vi "Left_to_Right_voltage.vi"(1 "left":dbl) -> (0 "right":dbl)   [LabVIEW 2009]
uses:
  <vilib>/gmath/NI_Gmath.lvlib
panel:
  in  "Left / Right Correlation":cluster{"right":dbl, "left":dbl}[](array[cluster])=[{"right"=0.0, "left"=0.0}, {"right"=0.52, "left"=0.5}, {"right"=0.79, "left"=0.75}, {"right"=1.02, "left"=1.0}, {"right"=1.27, "left"=1.25}, {"right"=1.52, "left"=1.5}, {"right"=1.77, "left"=1.75}, {"right"=2.0, "left"=2.0}, {"right"=2.25, "left"=2.25}, {"right"=2.5, "left"=2.5}, {"right"=2.75, "left"=2.75}, {"right"=3.0, "left"=3.0}, {"right"=3.23, "left"=3.25}, {"right"=3.48, "left"=3.5}, {"right"=3.71, "left"=3.75}, {"right"=3.96, "left"=4.0}, {"right"=4.22, "left"=4.25}, {"right"=4.45, "left"=4.5}, {"right"=4.56, "left"=4.75}, {"right"=4.58, "left"=5.0}]
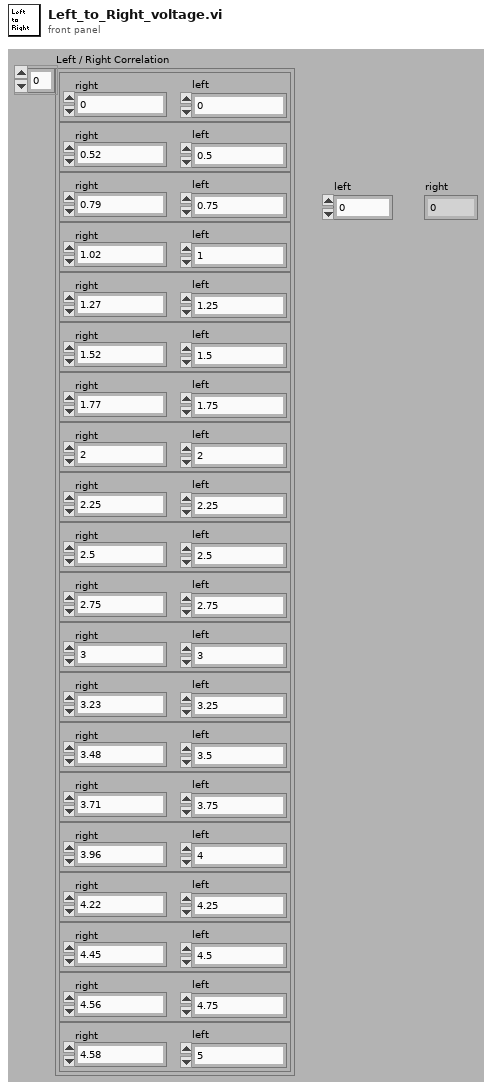
[diagram p1: front panel]
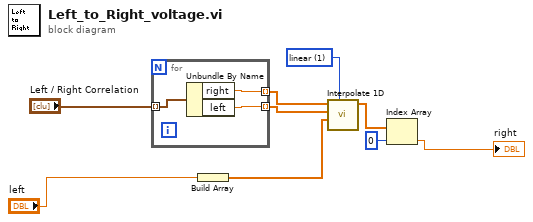
[diagram p0: block diagram]
diagram:
  w9 = 1 items=["nearest", "linear", "spline", "cubic Hermite", "Lagrange"] ("method")
  n1 = for {
    tunnel: "Left / Right Correlation" -> [w12] mode=indexing
    tunnel: [w11] -> w7 mode=indexing
    tunnel: [w10] -> w6 mode=indexing
    n2 = Unbundle By Name(w12) -> ("right"=w11:dbl, "left"=w10:dbl)
  }
  n3 = Build Array("left") -> (w1:dbl[])
  n4 = call <vilib>:"Interpolate 1D.vi"("method"=w9, "xi"=w1, "X"=w6, "Y"=w7) -> ("yi"=w5:dbl[])  [unwired: 5 in, 2 out]
  n5 = Index Array(array=w5, index=0) -> (element=→"right":dbl)
